vi "Set Top Level.vi"(8 "error in":errorcluster, 9 "Alias":string, 10 "Project Reference":refnum<vi>, 11 "VI Reference":refnum<vi>) -> (0 "error out":errorcluster)   [LabVIEW 2020]
doc: "Mark a VI in the project as the top level VI TopVI."
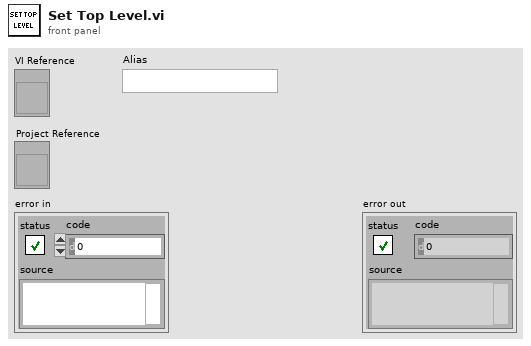
[diagram p1: front panel]
types:
  T1 = enum32{"invalid VI type", "Standard VI", "Control VI", "Global VI", "Polymorphic VI", "Configuration VI", "SubSystem", "Facade VI", "Method VI", "Statechart Diagram VI"}
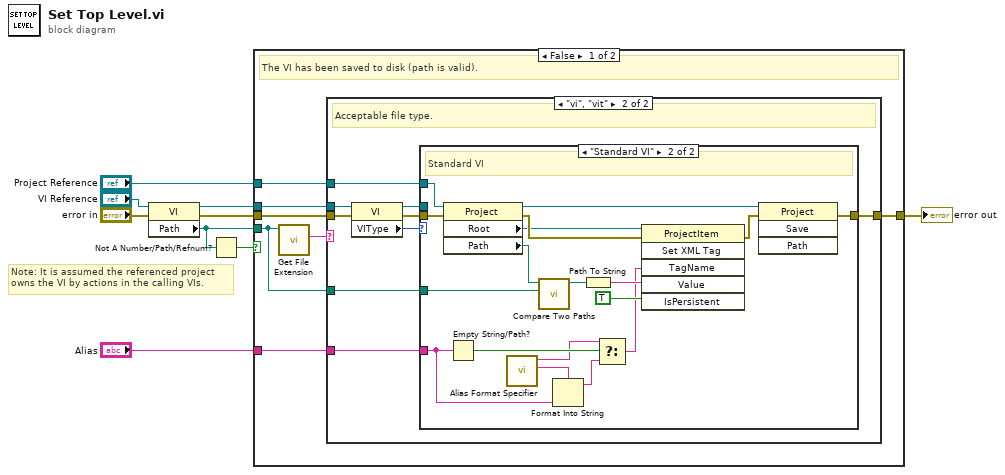
[diagram p0: block diagram]
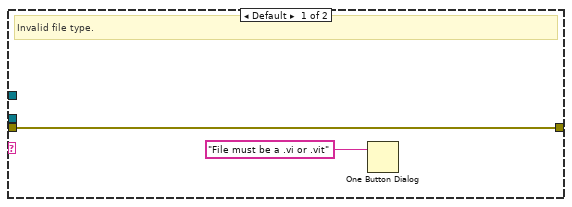
[diagram p2: hidden frame]
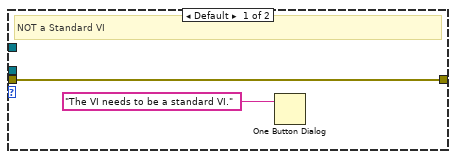
[diagram p3: hidden frame]
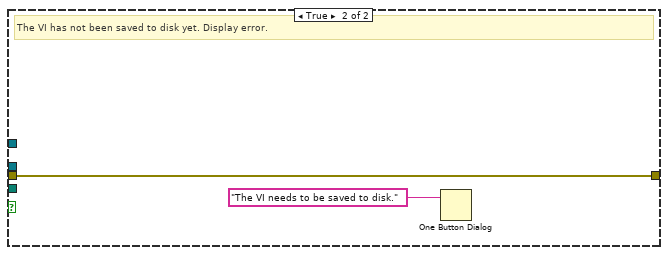
[diagram p4: hidden frame]
diagram:
  # "Note: It is assumed the referenced project owns the VI by actions in the calling VIs."
  n1 = property class="VI"(reference="VI Reference", error in="error in") -> (reference out=w2:refnum<vi>, error out=w7:errorcluster, "Path"=w5:path)
  n2 = Not A Number/Path/Refnum?(number/path/refnum=w5) -> (NaN/Path/Refnum?=w6:bool)
  n3 = case shown="False" w6 {
    tunnel: w7 -> [w16 w49]
    tunnel: [w15 w49] -> w9
    tunnel: w5 -> [w13 _]
    tunnel: "Project Reference" -> [w14 _]
    tunnel: w2 -> [w11 _]
    tunnel: "Alias" -> [w10 _]
    frame False {
      # "The VI has been saved to disk (path is valid)."
      n4 = call <vilib>:"Get File Extension.vi"("file"=w13) -> ("lowercase file extension"=w12:string)  [unwired: 6 in, 4 out]
      n5 = case shown="\"vi\", \"vit\"" w12 {
        tunnel: w16 -> [w18 w26]
        tunnel: [w18 w27] -> w15
        tunnel: w14 -> [_ w24]
        tunnel: w13 -> [_ w23]
        tunnel: w11 -> [_ w22]
        tunnel: w10 -> [_ w19]
        frame Default {
          # "Invalid file type."
          n6 = One Button Dialog(message="File must be a .vi or .vit") -> ()  [unwired: 1 in, 1 out]
        }
        frame "vi", "vit" {
          # "Acceptable file type."
          n7 = property class="VI"(reference=w22, error in=w26) -> (reference out=w20:refnum<vi>, error out=w25:errorcluster, "VIType"=w21:T1)
          n8 = case shown="\"Standard VI\"" w21 {
            tunnel: w25 -> [w29 w46]
            tunnel: [w29 w47] -> w27
            tunnel: w24 -> [_ w42]
            tunnel: w23 -> [_ w43]
            tunnel: w20 -> [_ _]
            tunnel: w19 -> [_ w30]
            frame Default {
              # "NOT a Standard VI"
              n9 = One Button Dialog(message="The VI needs to be a standard VI.") -> ()  [unwired: 1 in, 1 out]
            }
            frame "Standard VI" {
              # "Standard VI"
              n10 = property class="Project"(reference=w42, error in=w46) -> (reference out=w39:refnum<vi>, error out=w45:errorcluster, "Root"=w41:refnum<vi>, "Path"=w38:path)
              n11 = Empty String/Path?(string/path=w30) -> (empty?=w35:bool)
              n12 = call "Alias Format Specifier.vi"() -> ("Alias Format specifier"=w32:string, "Default Alias"=w31:string)  [unwired: 10 in]
              n13 = call <vilib>:"Compare Two Paths.vi"("Path 2"=w43, "Path 1"=w38) -> ("Relative Path from 1 to 2"=w37:path)  [unwired: 6 in, 3 out]
              n14 = Format Into String(format string=w32, w30) -> (resulting string=w34:string)  [unwired: 2 in, 1 out]
              n15 = Path To String(path=w37) -> (string=w36:string)
              n16 = Select(t=w31, s=w35, f=w34) -> (s? t:f=w33:string)
              n17 = invoke class="ProjectItem" method="Set XML Tag"(reference=w41, error in=w45, "TagName"=w33, "Value"=w36, "IsPersistent"=TRUE ("Is Persistent")) -> (error out=w44:errorcluster)  [unwired: 1 in, 5 out]
              n18 = invoke class="Project" method="Save"(reference=w39, error in=w44) -> (error out=w47:errorcluster)  [unwired: 2 in, 3 out]
            }
          }
        }
      }
    }
    frame True {
      # "The VI has not been saved to disk yet. Display error."
      n19 = One Button Dialog(message="The VI needs to be saved to disk.") -> ()  [unwired: 1 in, 1 out]
    }
  }
  "error out" <- w9
